vi "CreateNamesArray.vi"(11 "Cluster":T1) -> (3 "Array":string[](array[string]))   [LabVIEW 2014]
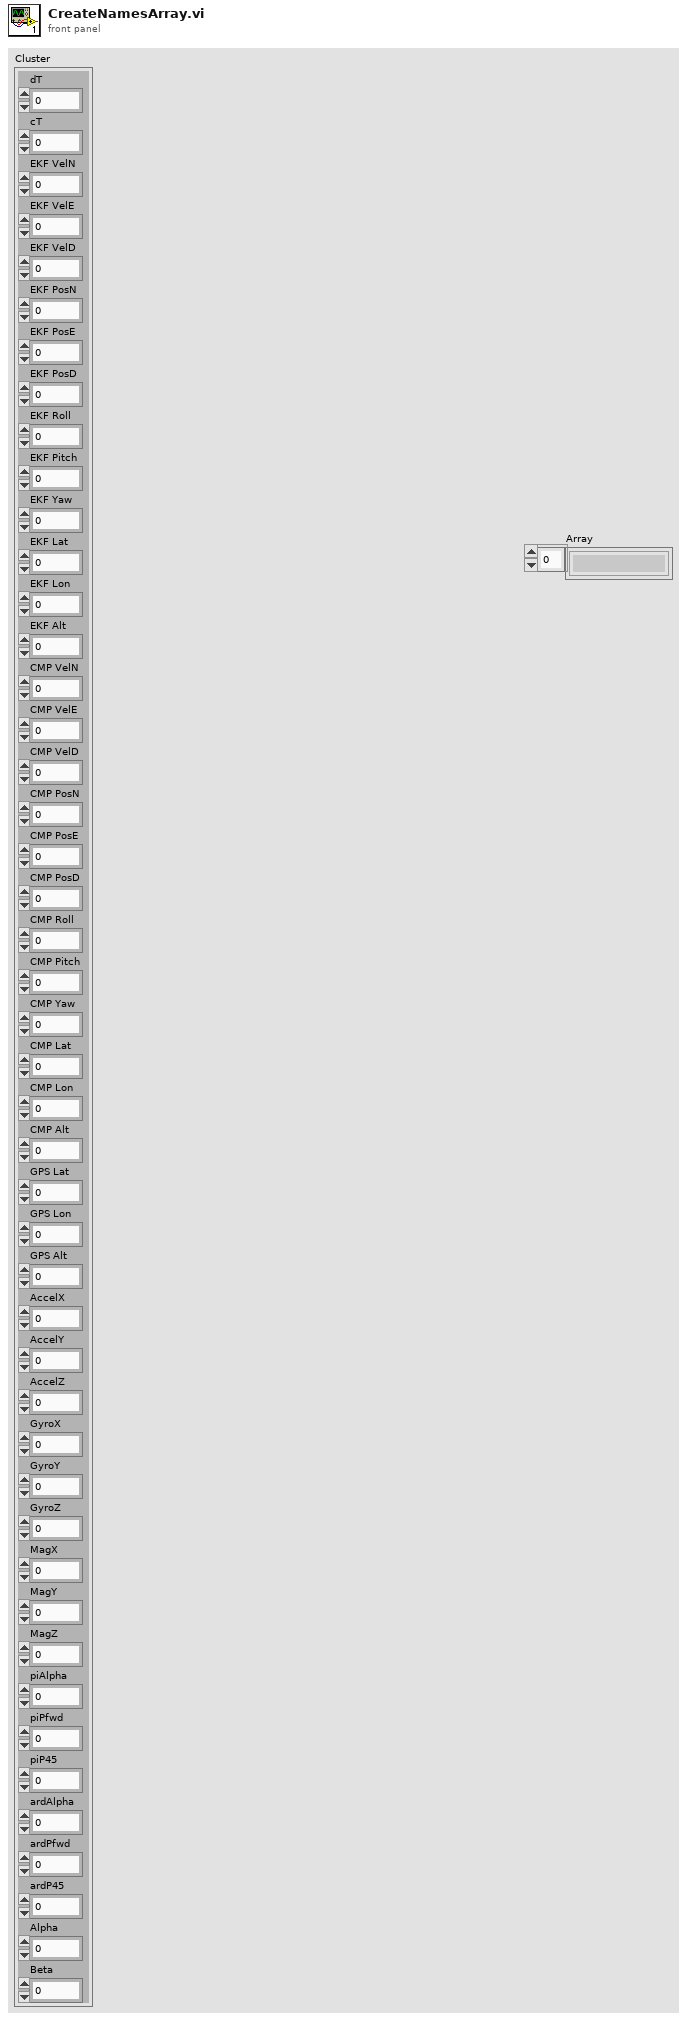
[diagram p1: front panel]
types:
  T1 = cluster{"dT":sgl, "cT":dbl, "EKF VelN":sgl, "EKF VelE":sgl, "EKF VelD":sgl, "EKF PosN":sgl, "EKF PosE":sgl, "EKF PosD":sgl, "EKF Roll":sgl, "EKF Pitch":sgl, "EKF Yaw":sgl, "EKF Lat":dbl, "EKF Lon":dbl, "EKF Alt":sgl, "CMP VelN":sgl, "CMP VelE":sgl, "CMP VelD":sgl, "CMP PosN":sgl, "CMP PosE":sgl, "CMP PosD":sgl, "CMP Roll":sgl, "CMP Pitch":sgl, "CMP Yaw":sgl, "CMP Lat":dbl, "CMP Lon":dbl, "CMP Alt":sgl, "GPS Lat":dbl, "GPS Lon":dbl, "GPS Alt":sgl, "AccelX":sgl, "AccelY":sgl, "AccelZ":sgl, "GyroX":sgl, "GyroY":sgl, "GyroZ":sgl, "MagX":sgl, "MagY":sgl, "MagZ":sgl, "piAlpha":sgl, "piPfwd":u16, "piP45":u16, "ardAlpha":sgl, "ardPfwd":u16, "ardP45":u16, "Alpha":sgl, "Beta":sgl}
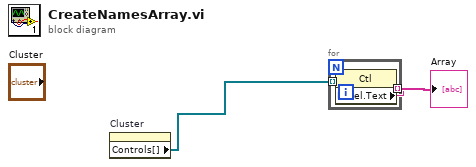
[diagram p0: block diagram]
diagram:
  n1 = property on="Cluster" class="Clust (strict)"() -> ("Controls[]"=w1:refnum<vi>[])  [unwired: 2 in, 2 out]
  n2 = for {
    tunnel: w1 -> [w4] mode=indexing
    tunnel: [w3] -> w2 mode=indexing
    n3 = property class="Ctl"(reference=w4) -> ("Label.Text"=w3:string)  [unwired: 1 in, 2 out]
  }
  "Array" <- w2
